vi "FRIC_navX_Get_Connect_Status.vi"(7 "Update":bool, 11 "Connected":bool) -> (3 "Connected":bool)   [LabVIEW 2015]
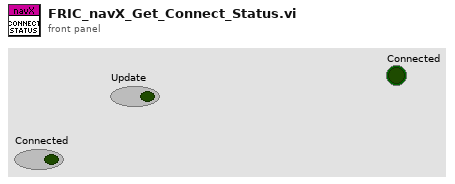
[diagram p1: front panel]
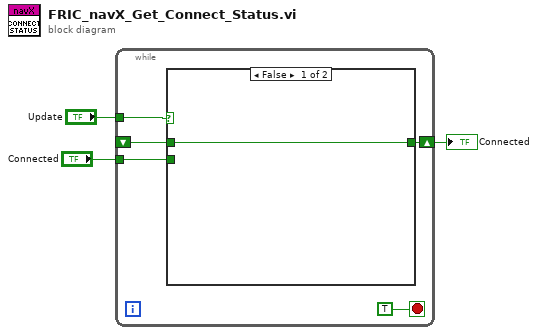
[diagram p0: block diagram]
diagram:
  n1 = while {
    tunnel: "Update" -> [w7]
    shift-right: [w4] -> w1
    shift-left: _ -> [w6]
    tunnel: "Connected" -> [w5]
    stop <- TRUE stop-if-true
    n2 = case shown="False" w7 {
      tunnel: w6 -> [w9 _]
      tunnel: w5 -> [_ w10]
      tunnel: [w9 w10] -> w4
      frame False {
      }
      frame True {
      }
    }
  }
  "Connected" <- w1
